vi "Read TC State Machine Setups.vi"(4 "Error In":errorcluster, 5 "Reload?":bool, 6 "Instance Name":T2, 7 "Config Data_Text in":refnum<class "Config Data_Text.lvclass">) -> (0 "Error Out":errorcluster, 2 "TC Parameters":T1, 3 "Config Data_Text out":refnum<class "Config Data_Text.lvclass">)   [LabVIEW 2015, in "Config Data.lvlib" / "Config Data_Text.lvclass"]
uses:
  Config Data_Text.lvclass
  Startup Processes/_typedefs/Subpanel Names.ctl
  Startup Processes/_typedefs/TC Setup Parameters.ctl
  <vilib>/Utility/config.llb/Read Key (String).vi
  <vilib>/Utility/config.llb/Write Key (String).vi
  <vilib>/Utility/config.llb/NI_LVConfig.lvlib
  Startup Processes/Startup Processes.lvlib
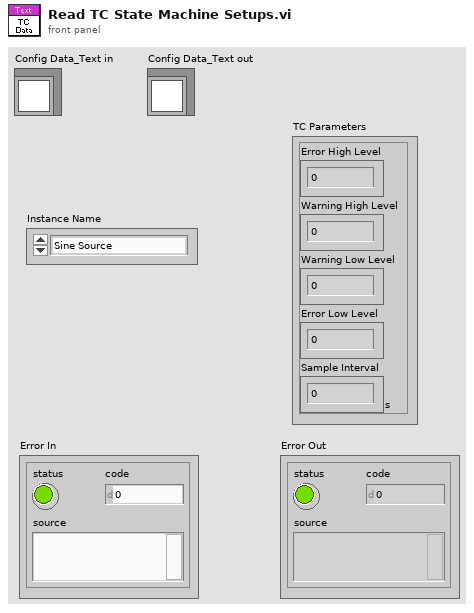
[diagram p1: front panel]
types:
  T1 = typedef "Startup Processes.lvlib/TC Setup Parameters.ctl" = cluster{"Error High Level":dbl, "Warning High Level":dbl, "Warning Low Level":dbl, "Error Low Level":dbl, "Sample Interval":dbl[unit]}
  T2 = typedef "Startup Processes.lvlib/Subpanel Names.ctl" = enum16{"Sine Source", "Ramp Source", "Hen House TC", "Dog House TC", "Out House TC"}
  T3 = cluster{"Error High Level":dbl, "Warning High Level":dbl, "Warning Low Level":dbl, "Error Low Level":dbl, "Sample Interval":dbl[unit]}
  T4 = typedef "NI_LVConfig.lvlib/Config Data RefNum.ctl" = refnum<k1>
  T5 = cluster{"Error High Level":dbl, "Warning High Level":dbl, "Warning Low Level":dbl, "Error Low Level":dbl, "Sample Interval":dbl[unit]}[]
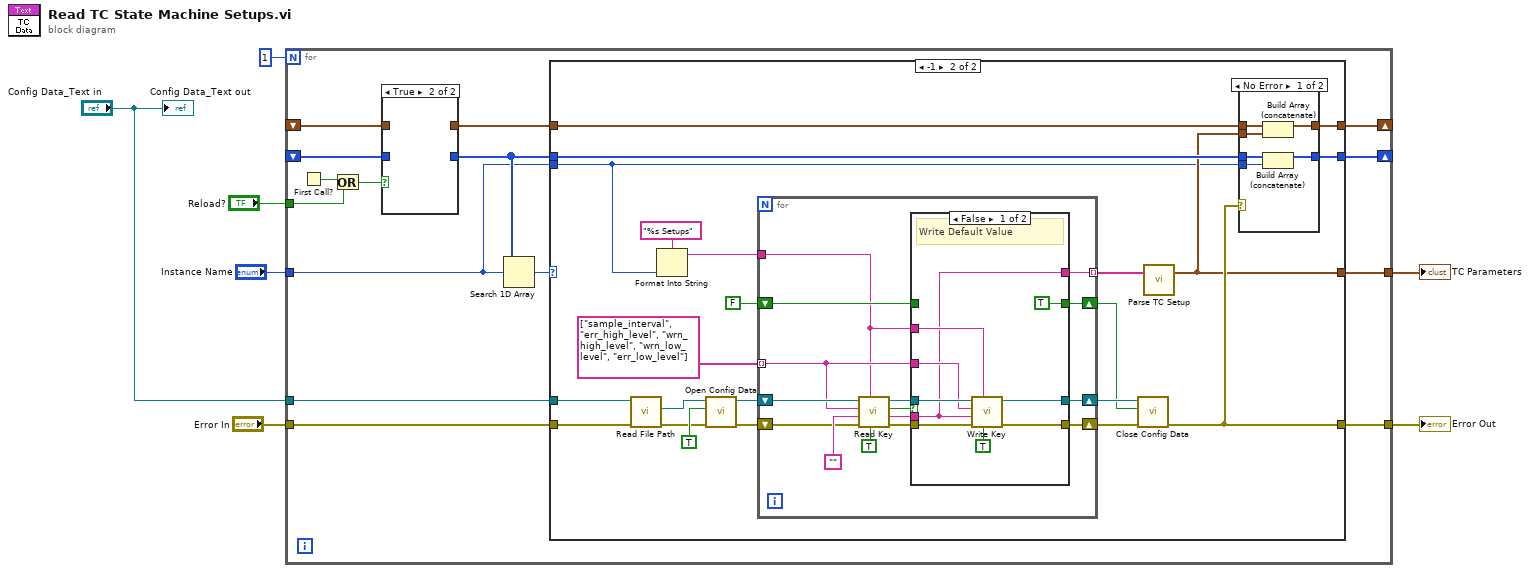
[diagram p0: block diagram]
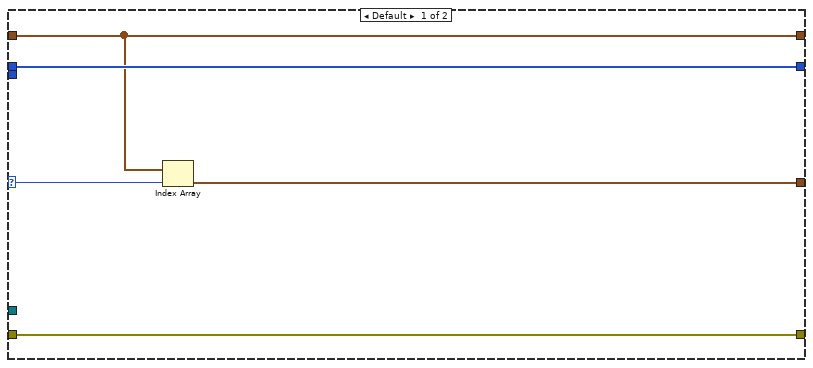
[diagram p3: hidden frame]
diagram:
  n1 = for {
    N: 1 -> [_]
    shift-right: [w18] -> _
    shift-left: _ -> [w17]
    shift-right: [w19] -> _
    shift-left: _ -> [w16]
    tunnel: "Error In" -> [w22]
    tunnel: [w21] -> w3
    tunnel: [w12] -> w4
    tunnel: "Instance Name" -> [w10]
    tunnel: "Config Data_Text in" -> [w11]
    tunnel: "Reload?" -> [w8]
    # "Read all Process VI definitions"
    n2 = First Call?() -> (First Call?: T/F=w15:bool)
    n3 = Or(x=w15, y=w8) -> (x .or. y?=w9:bool)
    n4 = case shown="True" w9 {
      tunnel: w17 -> [w23 _]
      tunnel: w16 -> [w24 _]
      tunnel: [w24 _] -> w14
      tunnel: [w23 _] -> w13
      frame False {
      }
      frame True {
      }
    }
    n5 = Search 1D Array(1D array=w14, element=w10) -> (index of element=w20:i32)  [unwired: 1 in]
    n6 = case shown="-1" w20 {
      selector: w20 -> [w25 _]
      tunnel: w22 -> [w28 w35]
      tunnel: [w28 w45] -> w21
      tunnel: w14 -> [w29 w49]
      tunnel: [w29 w48] -> w19
      tunnel: [w27 w47] -> w18
      tunnel: w13 -> [w27 w46]
      tunnel: w10 -> [_ w32]
      tunnel: [w26 w37] -> w12
      tunnel: w11 -> [_ w33]
      frame Default {
        n7 = Index Array(array=w27, index=w25) -> (element=w26:T3)
      }
      frame -1 {
        n8 = call "Read File Path.vi"("Error In"=w35, "Text In"=w33) -> ("Error Out"=w34:errorcluster, "File Path"=w36:path)  [unwired: 3 in, 1 out]
        n9 = Format Into String(format string="%s Setups" ("default value"), w32) -> (resulting string=w31:string)  [unwired: 2 in, 1 out]
        n10 = call <vilib>:"Open Config Data.vi"("error in (no error)"=w34, "create file if necessary (T)"=TRUE ("create file if necessary? (T)"), "configuration file path"=w36) -> ("error out"=w41:errorcluster, "refnum"=w40:T4)  [unwired: 6 in, 1 out]
        n11 = for {
          shift-right: [w59] -> w43
          shift-left: FALSE ("write configuration file? (T)") -> [w57]
          shift-right: [w61] -> w50
          shift-left: w40 -> [w55]
          shift-right: [w60] -> w44
          shift-left: w41 -> [w56]
          tunnel: string[] ["sample_interval", "err_high_level", "wrn_high_level", "wrn_low_level", "err_low_level"] -> [w53] mode=indexing
          tunnel: [w54] -> w38 mode=indexing
          tunnel: w31 -> [w52]
          n12 = call-poly <vilib>:"Read Key.vi"("read raw string? (F)"=TRUE, "section"=w52, "error in (no error)"=w56, "default value"="", "key"=w53, "refnum"=w55) -> ("error out"=w63:errorcluster, "value"=w62:string, "found?"=w65:bool, "refnum out"=w64:T4)  [unwired: 2 out]
          n13 = case shown="False" w65 {
            tunnel: w64 -> [w74 w78]
            tunnel: w52 -> [w73 _]
            tunnel: w63 -> [w75 w79]
            tunnel: [w70 w79] -> w60
            tunnel: [w71 w78] -> w61
            tunnel: w53 -> [w72 _]
            tunnel: w57 -> [_ w77]
            tunnel: [TRUE ("write configuration file? (T)") w77] -> w59
            tunnel: w62 -> [w67 w76]
            tunnel: [w67 w76] -> w54
            frame False {
              # "Write Default Value"
              n14 = call-poly <vilib>:"Write Key.vi"("write raw string? (F)"=TRUE ("read raw string? (F)"), "section"=w73, "error in (no error)"=w75, "value"=w67, "key"=w72, "refnum"=w74) -> ("error out"=w70:errorcluster, "refnum out"=w71:T4)  [unwired: 4 out]
            }
            frame True {
              # "Value Found"
            }
          }
        }
        n15 = call <vilib>:"Close Config Data.vi"("error in (no error)"=w44, "write file if changed (T)"=w43, "refnum"=w50) -> ("error out"=w45:errorcluster)  [unwired: 8 out]
        n16 = call "Parse TC Setup.vi"("INI File"=w38) -> ("TC Parameters"=w37:T3)  [unwired: 2 in]
        n17 = case shown="No Error" w45 {
          tunnel: w49 -> [w85 w86]
          tunnel: [w84 w86] -> w48
          tunnel: [w81 w87] -> w47
          tunnel: w46 -> [w82 w87]
          tunnel: w32 -> [w83 _]
          tunnel: w37 -> [w80 _]
          frame No Error {
            n18 = Build Array (concatenate)(w82, w80) -> (w81:T5)
            n19 = Build Array (concatenate)(w85, w83) -> (w84:T2[])
          }
          frame Error {
          }
        }
      }
    }
  }
  "Error Out" <- w3
  "TC Parameters" <- w4
  "Config Data_Text out" <- "Config Data_Text in"
